vi "Write FIFO (Four Channels).vi"(0 "data in":u32[](array[numeric]), 1 "enable":bool[](array[boolean]), 5 "input valid":bool, 8 "fifo 0":refnum<k21>, 9 "fifo 0 enable":bool, 11 "fifo 1 enable":bool, 12 "fifo 1":refnum<k21>, 13 "fifo 2 enable":bool, 14 "fifo 2":refnum<k21>, 15 "fifo 3 enable":bool, 16 "fifo 3":refnum<k21>) -> (17 "ready for input":bool)   [LabVIEW 2020]
doc: "Writes data to four 32-bit FIFOs. This VI is a wrapper around the LabVIEW FPGA FIFO Write method. This VI exposes handshaking signals that inform the user when the FIFOs are ready to accept new data.\n\n<B>Input Parameters</B>\n\n<B>data in</B> is the data to be written to the FIFO.\n\n<B>enabled</B> specifies which streams are enabled.\n\n<B>input valid</B> specifies when 'data in' is valid.\n\n<B>reset</B> the LabVIEW FPGA FIFO.\n\n<B>fifo 0</B> is the reference to the FIFO to which data received on channel 0 will be written to.\n\n<B>fifo 1</B> is the reference to the FIFO to which data received on channel 1 will be written to.\n\n<B>fifo 2</B> is the reference to the FIFO to which data received on channel 2 will be written to.\n\n<B>fifo 3</B> is the reference to the FIFO to which data received on channel 3 will be written to.\n\n<B>Output Parameters</B>\n\n<B>ready for input</B> is a flow control signal that indicates whether the Write FIFO VI is ready to accept new data."
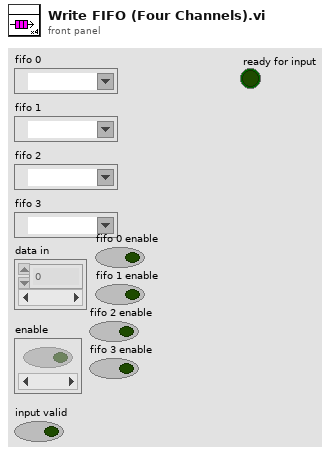
[diagram p1: front panel]
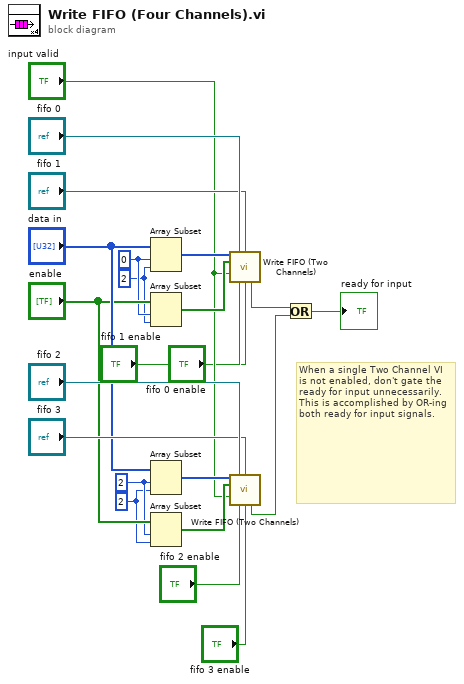
[diagram p0: block diagram]
diagram:
  w5 = 2 ("length")
  w6 = 2 ("index")
  w7 = 2 ("length")
  w8 = 0 ("index")
  # "When a single Two Channel VI is not enabled, don't gate the ready for input unnecessarily.  This is accomplished by OR-ing both ready for input signals."
  n1 = Array Subset(array="data in", index=w8, length=w7) -> (w15:u32[])
  n2 = Array Subset(array="enable", index=w8, length=w7) -> (w11:bool[])
  n3 = Array Subset(array="data in", index=w6, length=w5) -> (w13:u32[])
  n4 = Array Subset(array="enable", index=w6, length=w5) -> (w12:bool[])
  n5 = call "Write FIFO (Two Channels).vi"("data in"=w15, "fifo 0"="fifo 0", "fifo 1"="fifo 1", "enable"=w11, "input valid"="input valid", "fifo 0 enable"="fifo 0 enable", "fifo 1 enable"="fifo 1 enable") -> ("ready for input"=w18:bool)  [unwired: 8 in]
  n6 = call "Write FIFO (Two Channels).vi"("data in"=w13, "fifo 0"="fifo 2", "fifo 1"="fifo 3", "enable"=w12, "input valid"="input valid", "fifo 0 enable"="fifo 2 enable", "fifo 1 enable"="fifo 3 enable") -> ("ready for input"=w17:bool)  [unwired: 8 in]
  n7 = Or(x=w18, y=w17) -> (x .or. y?=→"ready for input":bool)
